vi "Run.vi"(7 "Team Index":i32, 8 "Column":i32, 9 "Row":i32, 10 "View":i32[](array[numeric]) caption="View (Team Index, -1: empty)", 11 "Awesome! In":refnum<class "Awesome!.lvclass">) -> (0 "Replicated":refnum<class "Square.lvclass">, 1 "Direction":T1, 2 "Action":T2, 3 "Square Out":refnum<class "Square.lvclass">)   [LabVIEW 2020, in "Awesome!.lvclass"]
uses:
  Awesome!.lvclass
  C:/dev/IlluminatedG/sol-squarebattle/Square/Square.lvclass
  Square/Square.lvclass
  Type Defs/Action Enum.ctl
  Type Defs/Direction Enum.ctl
  Awesome!.lvclass/Awesome!.ctl
  SubVIs/Globals (private).vi
  Common/Common.lvlib
  Type Defs/SB Type Defs.lvlib
  SubVIs/SB SubVIs.lvlib
panel:
  # "NW\nN\nNE\nE\nSE\nS\nSW\nW"
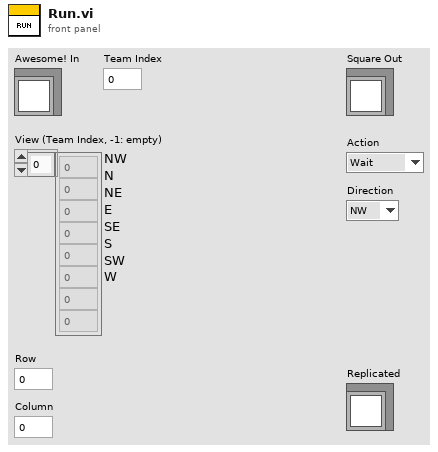
[diagram p1: front panel]
types:
  T1 = typedef "SB Type Defs.lvlib/Direction Enum.ctl" = enum16{"NW", "N", "NE", "E", "SE", "S", "SW", "W"}
  T2 = typedef "SB Type Defs.lvlib/Action Enum.ctl" = enum16{"Wait", "Move", "Attack", "Replicate"}
  T3 = typedef "Common.lvlib/Map DVR.ctl" = refnum<data-value>
  T4 = typedef "Common.lvlib/Position.ctl" = cluster{"Column":i32, "Row":i32}
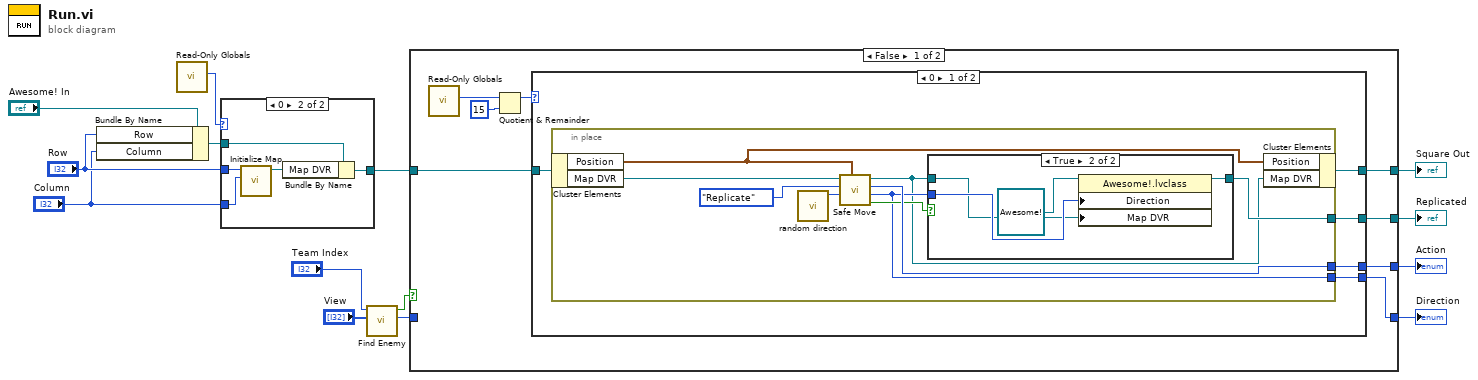
[diagram p0: block diagram]
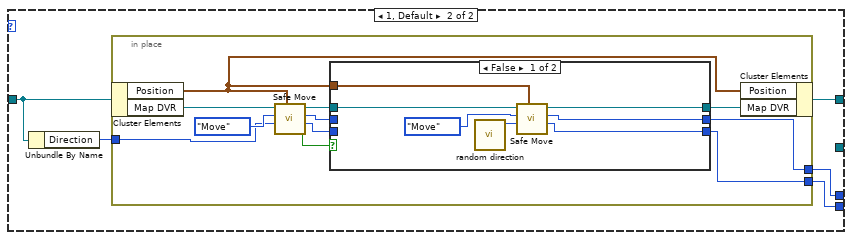
[diagram p4: hidden frame]
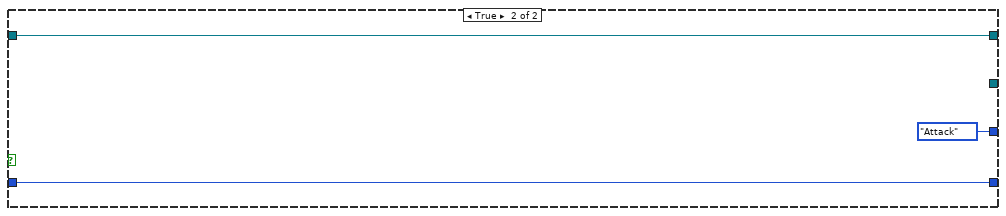
[diagram p6: hidden frame]
diagram:
  n1 = Bundle By Name(cluster="Awesome! In", "Row"="Row", "Column"="Column") -> (w4:refnum<class "Awesome!.lvclass">)
  n2 = call "Read-Only Globals.vi"() -> ("Round"=w6:i32)  [unwired: 10 in, 1 out]
  n3 = case shown="0" w6 {
    tunnel: w4 -> [w15 w17]
    tunnel: [w15 w16] -> w7
    tunnel: "Row" -> [_ w19]
    tunnel: "Column" -> [_ w18]
    frame Default {
    }
    frame 0 {
      n4 = call "Initialize Map.vi"("Column"=w18, "Row"=w19) -> ("Map DVR"=w20:T3)  [unwired: 9 in]
      n5 = Bundle By Name(cluster=w17, "Map DVR"=w20) -> (w16:refnum<class "Awesome!.lvclass">)
    }
  }
  n6 = call "Find Enemy.vi"("View"="View", "Team Index"="Team Index") -> ("Direction"=w11:T1, "Found Enemy?"=w14:bool)  [unwired: 7 in, 1 out]
  n7 = case shown="False" w14 {
    tunnel: w11 -> [_ w74]
    tunnel: [w25 Action_Enum."Attack" ("Action")] -> w10
    tunnel: [w23 w74] -> w9
    tunnel: w7 -> [w24 w73]
    tunnel: [w22 w73] -> w8
    tunnel: [w21 _] -> w1
    frame False {
      n8 = call "Read-Only Globals.vi"() -> ("Round"=w28:i32)  [unwired: 10 in, 1 out]
      n9 = Quotient & Remainder(x=w28, y=15) -> (x-y*floor(x/y)=w26:i32)  [unwired: 1 out]
      n10 = case shown="0" w26 {
        tunnel: [w31 w50] -> w25
        tunnel: w24 -> [w33 w48]
        tunnel: [w30 w49] -> w23
        tunnel: [w32 w51] -> w22
        tunnel: [w29 _] -> w21
        frame 0 {
          n11 = in-place {
            in-place-border: [w39] -> w31
            in-place-border: [w35] -> w30
            in-place-border: [w37] -> w29
            n12 = in-place-cluster #1(w33) -> ("Position"=w36:T4, "Map DVR"=w42:T3)
            n13 = call "random direction.vi"() -> ("Direction"=w40:T1)  [unwired: 11 in]
            n14 = call "Safe Move.vi"("Position in"=w36, "Direction in"=w40, "Desired Action"=Action_Enum."Replicate", "Map DVR"=w42) -> ("Accepted?"=w38:bool, "Direction"=w35:T1, "Action"=w39:T2, "Map DVR out"=w34:T3)  [unwired: 4 in]
            n15 = case shown="True" w38 {
              tunnel: w35 -> [_ w46]
              tunnel: [_ w44] -> w37
              tunnel: w34 -> [_ w43]
              frame False {
              }
              frame True {
                n16 = property class="Awesome!.lvclass"(reference=refnum<class "Awesome!.lvclass"> refnum ("Awesome!.lvclass"), "Direction"=w46, "Map DVR"=w43) -> (reference out=w44:refnum<class "Awesome!.lvclass">)  [unwired: 1 in, 1 out]
              }
            }
            n17 = in-place-cluster #1("Position"=w36, "Map DVR"=w34) -> (w32:refnum<class "Awesome!.lvclass">)
          }
        }
        frame 1, Default {
          n18 = Unbundle By Name(w48) -> ("Direction"=w47:T1)
          n19 = in-place {
            in-place-border: [w56] -> w50
            in-place-border: [w55] -> w49
            in-place-border: w47 -> [w52]
            n20 = in-place-cluster #2(w48) -> ("Position"=w57:T4, "Map DVR"=w62:T3)
            n21 = call "Safe Move.vi"("Position in"=w57, "Direction in"=w52, "Desired Action"=Action_Enum."Move" ("Action"), "Map DVR"=w62) -> ("Accepted?"=w60:bool, "Direction"=w53:T1, "Action"=w54:T2, "Map DVR out"=w59:T3)  [unwired: 4 in]
            n22 = case shown="False" w60 {
              tunnel: w59 -> [w69 w72]
              tunnel: [w68 w72] -> w58
              tunnel: w57 -> [w65 _]
              tunnel: [w64 w71] -> w56
              tunnel: [w63 w70] -> w55
              tunnel: w54 -> [_ w71]
              tunnel: w53 -> [_ w70]
              frame False {
                n23 = call "random direction.vi"() -> ("Direction"=w67:T1)  [unwired: 11 in]
                n24 = call "Safe Move.vi"("Position in"=w65, "Direction in"=w67, "Desired Action"=Action_Enum."Move", "Map DVR"=w69) -> ("Direction"=w63:T1, "Action"=w64:T2, "Map DVR out"=w68:T3)  [unwired: 4 in, 1 out]
              }
              frame True {
              }
            }
            n25 = in-place-cluster #2("Position"=w57, "Map DVR"=w58) -> (w51:refnum<class "Awesome!.lvclass">)
          }
        }
      }
    }
    frame True {
    }
  }
  "Square Out" <- w8
  "Action" <- w10
  "Direction" <- w9
  "Replicated" <- w1
